vi "Sine Fit Model.vi"(6 "Ignore Offset":bool, 9 "Length":i32, 10 "Sample Rate":i32, 11 "Frequency":dbl) -> (3 "Array":ext[][](array[numeric]))   [LabVIEW 2016, in "Sinusoidal Fit.lvclass"]
uses:
  Sinusoidal Fit.lvclass
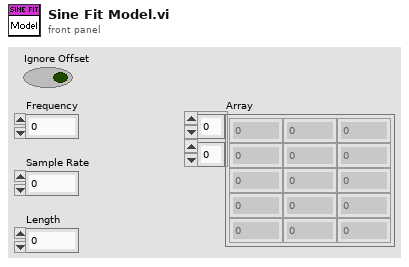
[diagram p1: front panel]
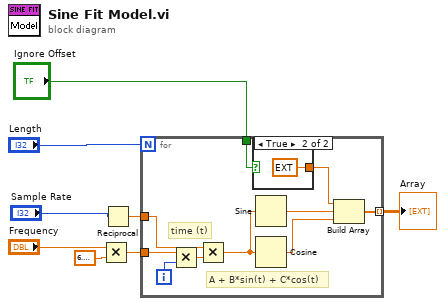
[diagram p0: block diagram]
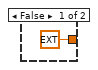
[diagram p2: hidden frame]
diagram:
  n1 = Multiply(x="Frequency", y=6.283185307179586) -> (x*y=w5:dbl)
  n2 = Reciprocal(x="Sample Rate") -> (1/x=w2:dbl)
  n3 = for {
    N: "Length" -> [_]
    tunnel: w5 -> [w18]
    tunnel: [w11] -> w6 mode=indexing
    tunnel: w2 -> [w10]
    tunnel: "Ignore Offset" -> [w9]
    i -> [w17]
    # "A + B*sin(t) + C*cos(t)"
    # "time (t)"
    n4 = Multiply(x=w18, y=w17) -> (x*y=w16:dbl)
    n5 = Multiply(x=w10, y=w16) -> (x*y=w15:dbl)
    n6 = case shown="True" w9 {
      tunnel: [ext 1.0 ("Input Element") ext 0.0 ("Input Element")] -> w12
      frame False {
      }
      frame True {
      }
    }
    n7 = Sine(x=w15) -> (sin(x)=w13:dbl)
    n8 = Cosine(x=w15) -> (cos(x)=w14:dbl)
    n9 = Build Array(w12, w13, w14) -> (w11:ext[])
  }
  "Array" <- w6
